vi "Generate.vi"(8 "error in (no error)":errorcluster, 10 "Data Notifier":refnum<notifier>, 11 "Hardware Resources in":T1={"AO"={"task name"="AO", "task_ref"="", "physical channels"="Dev1/ao0"}, "PID"={"P"=0.0, "I"=0.0, "D"=0.0}, "conversions"={"ao0"={"a"=0.0, "b"=0.0}}, "setpoint"=0.0}) -> (0 "error out":errorcluster, 3 "Hardware Resources out":T1={"AO"={"task name"="AO", "task_ref"="", "physical channels"="Dev1/ao0"}, "PID"={"P"=0.0, "I"=0.0, "D"=0.0}, "conversions"={"ao0"={"a"=0.0, "b"=0.0}}, "setpoint"=0.0})   [LabVIEW 2014, in "PLS Generation.lvlib"]
doc: "Perform the acquisition. Replace the contents of this diagram with calls to acquisition hardware."
uses:
  PLS Generation.lvlib
  Hardware Configuration.ctl
  Settings/conversion.ctl
  <vilib>/DAQmx/write.llb/DAQmx Write (Analog DBL 1Chan 1Samp).vi
  <vilib>/addons/control/pid/pid.llb/PID (DBL).vi
  <vilib>/DAQmx/miscellaneous.llb/DAQmx Fill In Error Info.vi
  <vilib>/addons/control/pid/NI_PID_pid.lvlib
  Settings/PLS Settings.lvlib
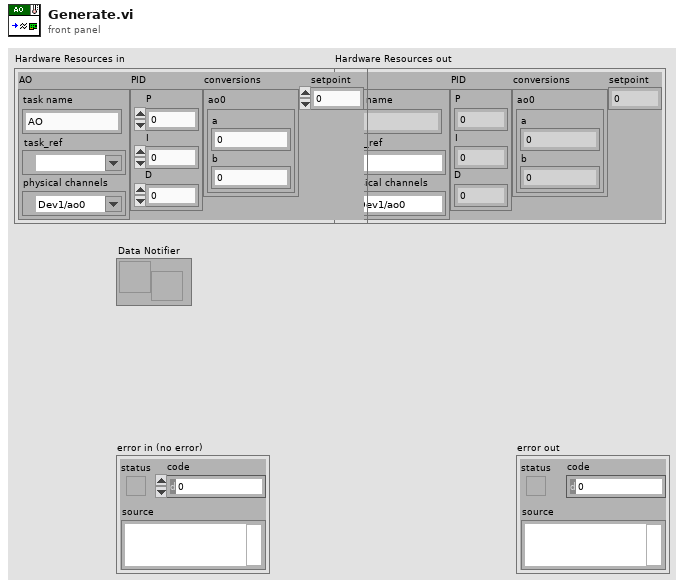
[diagram p1: front panel]
types:
  T1 = typedef "PLS Generation.lvlib/Hardware Configuration.ctl" = cluster{"AO":cluster{"task name":string, "task_ref":refnum<k21>, "physical channels":tag}, "PID":cluster{"P":dbl, "I":dbl, "D":dbl}, "conversions":cluster{"ao0":T2}, "setpoint":dbl}
  T2 = typedef "PLS Settings.lvlib/conversion.ctl" = cluster{"a":dbl, "b":dbl}
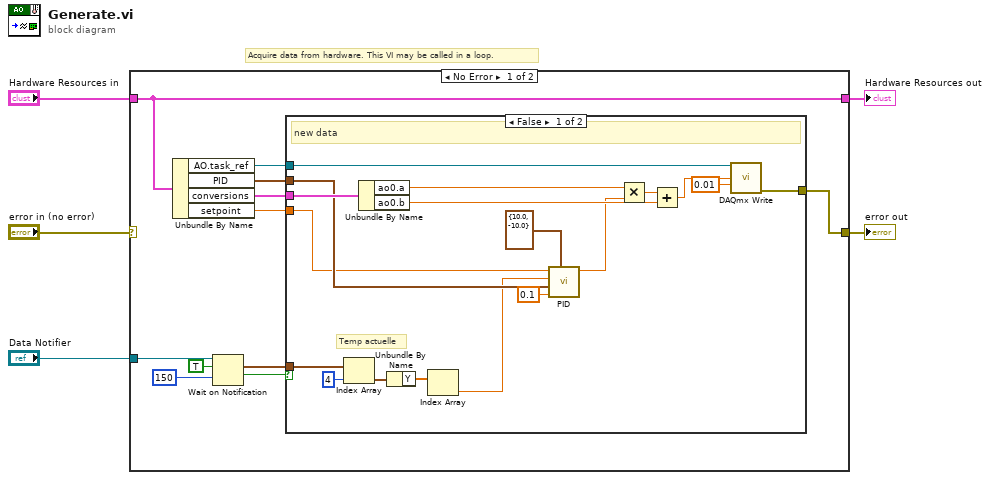
[diagram p0: block diagram]
diagram:
  # "Acquire data from hardware. This VI may be called in a loop."
  n1 = case shown="No Error" "error in (no error)" {
    selector: "error in (no error)" -> [_ w35]
    tunnel: [w7 w35] -> w4
    tunnel: "Hardware Resources in" -> [w16 w36]
    tunnel: [w16 w36] -> w2
    tunnel: "Data Notifier" -> [w15 _]
    frame No Error {
      n2 = Unbundle By Name(w16) -> ("AO.task_ref"=w11:refnum<k21>, "PID"=w10:cluster{"P":dbl, "I":dbl, "D":dbl}, "conversions"=w8:cluster{"ao0":T2}, "setpoint"=w6:dbl)
      n3 = Wait on Notification(notifier=w15, ignore previous (F)=TRUE, timeout in ms (-1)=150) -> (notification=w9:waveform(dbl)[], timed out?=w12:bool)  [unwired: 1 in, 2 out]
      n4 = case shown="False" w12 {
        tunnel: w11 -> [w31 _]
        tunnel: w10 -> [w22 _]
        tunnel: w9 -> [w34 _]
        tunnel: w8 -> [w28 _]
        tunnel: [w29 _] -> w7
        tunnel: w6 -> [w19 _]
        frame False {
          # "Temp actuelle"
          # "new data"
          n5 = Index Array(array=w34, index=4) -> (element=w33:waveform(dbl))
          n6 = Unbundle By Name(w28) -> ("ao0.a"=w27:dbl, "ao0.b"=w25:dbl)
          n7 = Unbundle By Name(w33) -> ("Y"=w32:dbl[])
          n8 = Index Array(array=w32) -> (element=w20:dbl)  [unwired: 1 in]
          n9 = call-poly <vilib>:"PID.vi"("output range"=cluster{"output high":dbl, "output low":dbl} {"output high"=10.0, "output low"=-10.0}, "dt (s)"=0.1, "PID gains"=w22, "process variable"=w20, "setpoint"=w19) -> ("output"=w21:dbl)  [unwired: 5 in, 1 out]
          n10 = Multiply(x=w27, y=w21) -> (x*y=w26:dbl)
          n11 = Add(x=w26, y=w25) -> (x+y=w24:dbl)
          n12 = call-poly <vilib>:"DAQmx Write.vi"("task/channels in"=w31, "data"=w24, "timeout"=0.01) -> ("error out"=w29:errorcluster)  [unwired: 10 in, 2 out]
        }
        frame True {
          # "timeout - no new data"
        }
      }
    }
    frame Error {
    }
  }
  "Hardware Resources out" <- w2
  "error out" <- w4
